vi "Temp input.vi"() -> (0 "Array":dbl[](array[numeric]))   [LabVIEW 2015]
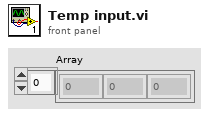
[diagram p1: front panel]
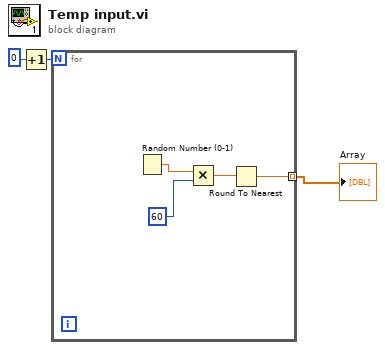
[diagram p0: block diagram]
diagram:
  n1 = Increment(x=0) -> (x+1=w3:i32)
  n2 = for {
    N: w3 -> [_]
    tunnel: [w4] -> w1 mode=indexing
    n3 = Random Number (0-1)() -> (number: 0 to 1=w7:dbl)
    n4 = Multiply(x=w7, y=60) -> (x*y=w5:dbl)
    n5 = Round To Nearest(number=w5) -> (nearest integer value=w4:dbl)
  }
  "Array" <- w1
